vi "Set Dynamic Dispatch.vi"(8 "error in (no error)":errorcluster, 10 "Dynamic?":bool, 11 "VI Refnum In":refnum<vi>) -> (0 "error out":errorcluster, 3 "VI Refnum":refnum<vi>)   [LabVIEW 2018, in "LVClassByRef.lvlib"]
uses:
  <resource>/Framework/Providers/LVClassByRef/LVClassByRef.lvlib
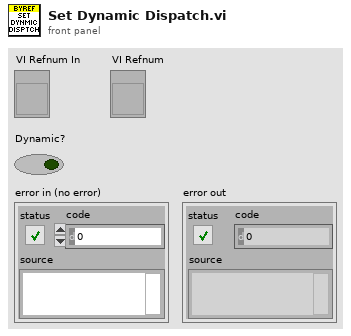
[diagram p1: front panel]
types:
  T1 = enum16{"Invalid Wire Rule", "Required", "Recommended", "Optional", "Dynamic Dispatch"}
  T2 = enum16{"Invalid Wire Rule", "Required", "Recommended", "Optional", "Dynamic Dispatch"}[]
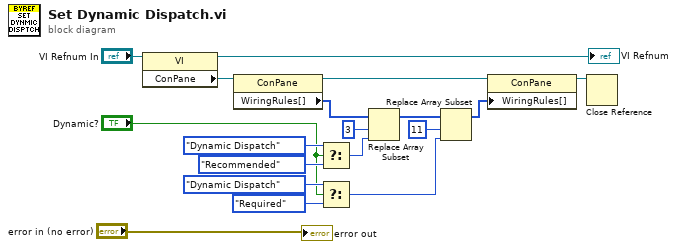
[diagram p0: block diagram]
diagram:
  n1 = property class="VI"(reference="VI Refnum In") -> (reference out=→"VI Refnum":refnum<vi>, "ConPane"=w17:refnum<vi>)  [unwired: 1 in, 1 out]
  n2 = property class="ConPane"(reference=w17) -> (reference out=w4:refnum<vi>, "WiringRules[]"=w16:T2)  [unwired: 1 in, 1 out]
  n3 = Select(t=T1."Dynamic Dispatch" ("new element/subarray"), s="Dynamic?", f=T1."Recommended") -> (s? t:f=w10:T1)
  n4 = Select(t=T1."Dynamic Dispatch" ("new element/subarray"), s="Dynamic?", f=T1."Required") -> (s? t:f=w7:T1)
  n5 = Replace Array Subset(array=w16, new element=w10, index=3) -> (w15:T2)
  n6 = Replace Array Subset(array=w15, new element=w7, index=11) -> (w5:T2)
  n7 = property class="ConPane"(reference=w4, "WiringRules[]"=w5) -> (reference out=w3:refnum<vi>)  [unwired: 1 in, 1 out]
  n8 = Close Reference(reference=w3) -> ()  [unwired: 1 in, 1 out]
  "error out" <- "error in (no error)"
